vi "Two Color Cal Get Image.vi"(0 "Notifier Name":string, 7 "Write File Ref":refnum<file>, 11 "Num of Frames":u16) -> ()   [LabVIEW 2016]
uses:
  Device Library/Cameras/Camera Controls/Generic Camera Actions.ctl
  Device Library/Cameras/Camera Controls/Camera IMAQ Key Info.ctl
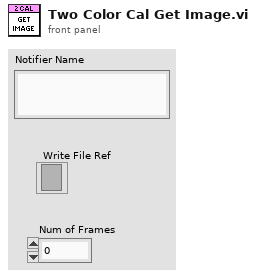
[diagram p1: front panel]
types:
  T1 = typedef "Generic Camera Actions.ctl" = enum16{"Status", "Live Preview", "Capture", "Abort", "Set Exposure Time (s)", "Get Exposure Time (s)", "Record Settings", "Set ROI", "Get ROI", "Defect Correction On/Off", "Cooler On/Off", "Fan On/Off", "Quti"}
  T2 = typedef "IMAQ Image.ctl" = refnum<image>
  T3 = enum16{"big-endian, network order", "native, host order", "little-endian"}
  T4 = typedef "Camera IMAQ Key Info.ctl" = cluster{"Frame":u32, "Sensor Height":i32, "Sensor Width":i32, "ROI Height":i32, "ROI Width":i32, "ROI Enable?":bool, "Bit per Pixel":u8}
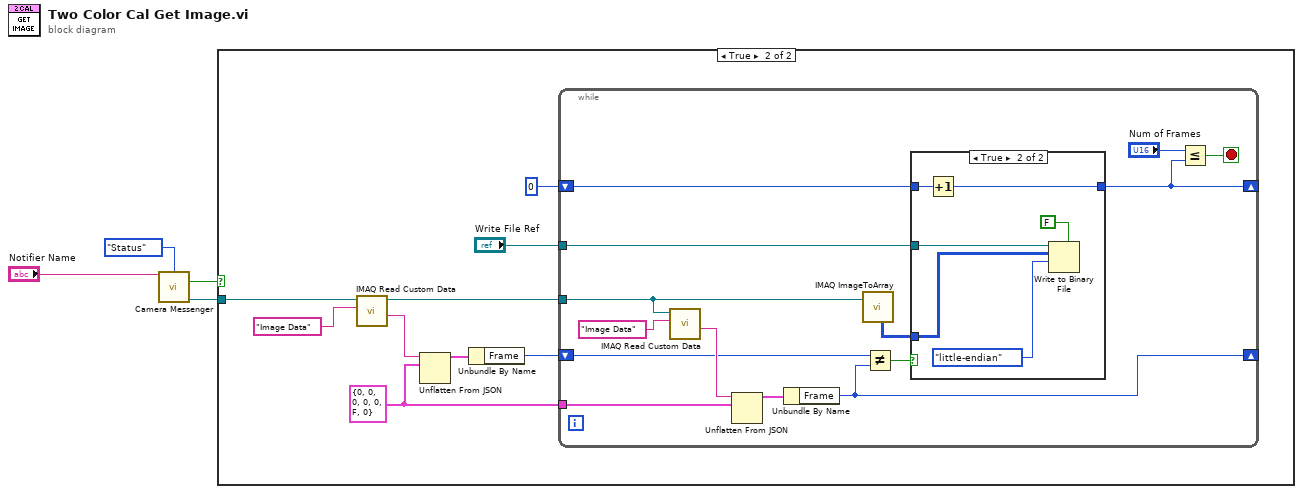
[diagram p0: block diagram]
diagram:
  n1 = call "Camera Messenger.vi"("Notifier Name"="Notifier Name", "General Camera Actions"=Generic_Camera_Actions."Status") -> ("Running?"=w1:bool, "Image Ref"=w3:T2)  [unwired: 8 in, 4 out]
  n2 = case shown="True" w1 {
    tunnel: w3 -> [_ w11]
    frame False {
    }
    frame True {
      w8 = T4 {"Frame"=0, "Sensor Height"=0, "Sensor Width"=0, "ROI Height"=0, "ROI Width"=0, "ROI Enable?"=FALSE, "Bit per Pixel"=0} ("Camera IMAQ Key Info")
      n3 = call "IMAQ Read Custom Data"("Key"="Image Data", "Image"=w11) -> ("Custom Data Out"=w13:string, "Image (duplicate)"=w7:T2)  [unwired: 7 in, 1 out]
      n4 = Unflatten From JSON(JSON string=w13, type and defaults=w8) -> (value=w10:T4)  [unwired: 5 in, 1 out]
      n5 = Unbundle By Name(w10) -> ("Frame"=w9:u32)
      n6 = while {
        tunnel: w7 -> [w22]
        shift-right: [w17] -> _
        shift-left: w9 -> [w23]
        tunnel: w8 -> [w24]
        shift-right: [w16] -> _
        shift-left: u16 0 ("element") -> [w19]
        tunnel: "Write File Ref" -> [w18]
        stop <- w15 stop-if-true
        n7 = call "IMAQ Read Custom Data"("Key"="Image Data", "Image"=w22) -> ("Custom Data Out"=w26:string)  [unwired: 7 in, 2 out]
        n8 = Unflatten From JSON(JSON string=w26, type and defaults=w24) -> (value=w27:T4)  [unwired: 5 in, 1 out]
        n9 = Unbundle By Name(w27) -> ("Frame"=w17:u32)
        n10 = call "IMAQ ImageToArray"("Image"=w22) -> ("Image Pixels (U16)"=w20:u16[][])  [unwired: 3 in, 4 out]
        n11 = Not Equal?(x=w23, y=w17) -> (x != y?=w21:bool)
        n12 = case shown="True" w21 {
          tunnel: w20 -> [_ w30]
          tunnel: w19 -> [w28 w34]
          tunnel: [w28 w33] -> w16
          tunnel: w18 -> [_ w31]
          frame False {
          }
          frame True {
            n13 = Increment(x=w34) -> (x+1=w33:u16)
            n14 = Write to Binary File(file (use dialog)=w31, data=w30, 5:FALSE ("prepend array or string size? (T)"), 9:T3."little-endian" ("byte order (0:big-endian, network order)")) -> ()  [unwired: 2 in, 3 out]
          }
        }
        n15 = Less Or Equal?(x="Num of Frames", y=w16) -> (x <= y?=w15:bool)
      }
    }
  }
